vi "get_config_cluster.vi"(8 "error in (no error)":errorcluster, 11 "GenericPlugin in":refnum<class "SignalReaderCN091129DAQmx.lvclass">) -> (0 "error out":errorcluster, 2 "config cluster (variant)":variant, 3 "GenericPlugin out":refnum<class "SignalReaderCN091129DAQmx.lvclass">)   [LabVIEW 2010, in "SignalReaderCN091129DAQmx.lvclass"]
uses:
  SignalReaderCN091129DAQmx.lvclass
  SignalReaderCN091129DAQmx.lvclass/SignalReaderCN091129DAQmx.ctl
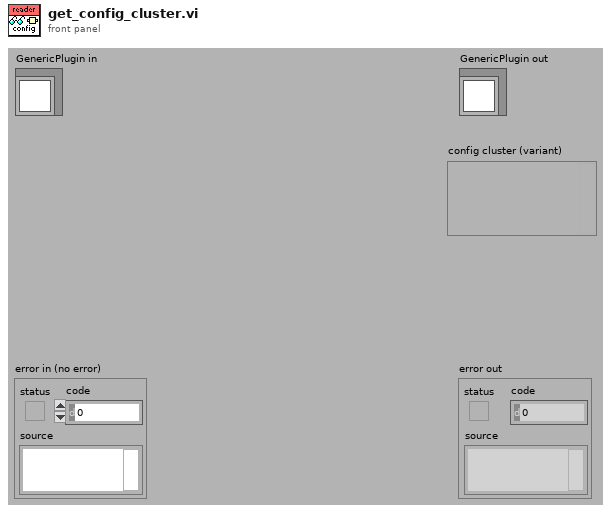
[diagram p1: front panel]
types:
  T1 = typedef "SignalReaderCN091129DAQmx.lvclass/config_data_cluster.ctl" = cluster{"analog input channels":T2[], "clock source":string, "time-out":dbl[unit], "maximum sampling rate":dbl[unit], "buffer size":i32}
  T2 = typedef "SignalReaderCN091129DAQmx.lvclass/channel_definition_cluster.ctl" = cluster{"physical Channel":string, "max_input_value":dbl, "min_input_value":dbl, "ground_reference":i32, "translation_factor":dbl, "translation_offset":dbl}
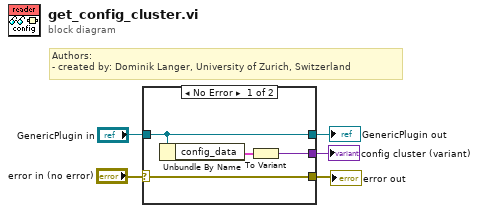
[diagram p0: block diagram]
diagram:
  # "Authors: \n- created by: Dominik Langer, University of Zurich, Switzerland"
  n1 = case shown="No Error" "error in (no error)" {
    selector: "error in (no error)" -> [w9 w10]
    tunnel: "GenericPlugin in" -> [w8 w11]
    tunnel: [w9 w10] -> w2
    tunnel: [w8 w11] -> w1
    tunnel: [w6 _] -> w3
    frame No Error {
      n2 = Unbundle By Name(w8) -> ("config_data"=w7:T1)
      n3 = To Variant(anything=w7) -> (Variant=w6:variant)
    }
    frame Error {
    }
  }
  "error out" <- w2
  "GenericPlugin out" <- w1
  "config cluster (variant)" <- w3
